vi "Render.vi"(8 "error in":errorcluster, 10 "Renderer in":refnum<class "Renderer.lvclass">, 11 "Dqmh Module":refnum<class "Dqmh Module.lvclass">) -> (0 "error out":errorcluster, 3 "Sections out":refnum<class "Section.lvclass">[](array[class]))   [LabVIEW 2021, in "TAF Proj Document Type.lvlib" / "Dqmh Module.lvclass"]
uses:
  <vilib>/Wovalab/AntiDoc/Document Type/Add-ons/LabVIEW TAF Project/Dqmh Module/Dqmh Module.lvclass
  C:/Program Files (x86)/National Instruments/LabVIEW 2021/vi.lib/Wovalab/AntiDoc/Bloc/Bloc.lvclass
  C:/Program Files (x86)/National Instruments/LabVIEW 2021/vi.lib/Wovalab/AntiDoc/Document Type/Add-ons/LabVIEW TAF Project/Lib/Lib.lvclass
  <vilib>/Wovalab/AntiDoc/Renderer/Renderer.lvclass
  <vilib>/Wovalab/AsciiDoc for LabVIEW/Section/Section.lvclass
  <vilib>/Wovalab/AsciiDoc for LabVIEW/Diagram/Type--enum.ctl
  <vilib>/Wovalab/AntiDoc/Document Type/Add-ons/LabVIEW TAF Project/Dqmh Module/Event Callers--cluster.ctl
  <vilib>/Wovalab/AsciiDoc for LabVIEW/Admonition/Types--enum.ctl
  <vilib>/Wovalab/AsciiDoc for LabVIEW/Table/Column Attributes--cluster.ctl
  <vilib>/Wovalab/AsciiDoc for LabVIEW/Table/Horizontal Alignment--enum.ctl
  <vilib>/Wovalab/AsciiDoc for LabVIEW/Table/Vertical Alignment--enum.ctl
  <vilib>/Wovalab/AsciiDoc for LabVIEW/Table/Style--enum.ctl
  <vilib>/Wovalab/AntiDoc/Bloc/Bloc.lvclass/Bloc.ctl
  <vilib>/Wovalab/AntiDoc/Document Type/Add-ons/LabVIEW TAF Project/Dqmh Module/Dqmh Module.lvclass/Dqmh Module.ctl
  <vilib>/Wovalab/AntiDoc/Document Type/Add-ons/LabVIEW TAF Project/Lib/Lib.lvclass/Lib.ctl
  <vilib>/Wovalab/AntiDoc/Renderer/Renderer.lvclass/Renderer.ctl
  <vilib>/Wovalab/AsciiDoc for LabVIEW/Table/Table.lvclass/Table.ctl
  <vilib>/Wovalab/AntiDoc/Renderer/Read Image Folder Path.vi
  <vilib>/Wovalab/AntiDoc/Bloc/Read Name.vi
  <vilib>/Wovalab/AntiDoc/Document Type/Add-ons/LabVIEW TAF Project/Dqmh Module/Read Dqmh Module Type.vi
  <vilib>/Wovalab/AntiDoc/Document Type/Add-ons/LabVIEW TAF Project/Lib/Read Description.vi
  <vilib>/Wovalab/AntiDoc/Document Type/Add-ons/LabVIEW TAF Project/Dqmh Module/Read Start Module Callers.vi
  <vilib>/Wovalab/AntiDoc/Document Type/Add-ons/LabVIEW TAF Project/Dqmh Module/Read Stop Module Callers.vi
  <vilib>/Wovalab/AntiDoc/Document Type/Add-ons/LabVIEW TAF Project/Dqmh Module/Read Request Link.vi
  <vilib>/Wovalab/AntiDoc/Document Type/Add-ons/LabVIEW TAF Project/Dqmh Module/Read Request With Reply Links.vi
  <vilib>/Wovalab/AntiDoc/Document Type/Add-ons/LabVIEW TAF Project/Dqmh Module/Read Broadcast Link.vi
  <vilib>/Wovalab/AntiDoc/Document Type/Add-ons/LabVIEW TAF Project/Dqmh Module/Read Registred Broadcast.vi
  <vilib>/Wovalab/AntiDoc/Document Type/Add-ons/LabVIEW TAF Project/Dqmh Module/Read Used Requests.vi
  <vilib>/Wovalab/AntiDoc/Document Type/Add-ons/LabVIEW TAF Project/Dqmh Module/Read Used Requests With Reply.vi
  <vilib>/Wovalab/AntiDoc/Document Type/Add-ons/LabVIEW TAF Project/Dqmh Module/Read Custom Errors.vi
  <vilib>/Wovalab/AntiDoc/Document Type/Add-ons/LabVIEW TAF Project/Lib/Read Vis.vi
  <vilib>/Wovalab/AntiDoc/Document Type/Add-ons/LabVIEW TAF Project/Dqmh Module/Read List Default Event.vi
  <vilib>/Wovalab/AsciiDoc for LabVIEW/Paragraph/Paragraph.lvclass
  C:/Program Files (x86)/National Instruments/LabVIEW 2021/vi.lib/Wovalab/AsciiDoc for LabVIEW/Adoc-Bloc/Bloc.lvclass
  <vilib>/Wovalab/AsciiDoc for LabVIEW/Admonition/Admonition.lvclass
  <vilib>/Wovalab/AsciiDoc for LabVIEW/Table/Table.lvclass
  <vilib>/Wovalab/AsciiDoc for LabVIEW/Diagram/Diagram.lvclass
  <vilib>/Wovalab/AsciiDoc for LabVIEW/Sub Section/Sub Section.lvclass
  C:/Program Files (x86)/National Instruments/LabVIEW 2021/vi.lib/Wovalab/AsciiDoc for LabVIEW/Section/Section.lvclass
  <vilib>/Wovalab/AsciiDoc for LabVIEW/Section/Add Bloc (array).vi
  <vilib>/Wovalab/AsciiDoc for LabVIEW/Sub Section/Create Sub Section (array).vi
  <vilib>/Wovalab/AntiDoc/Document Type/Add-ons/LabVIEW TAF Project/Vi/Vi.lvclass
  <vilib>/Wovalab/AntiDoc/Utilities/Utilities.lvlib
  C:/Program Files (x86)/National Instruments/LabVIEW 2021/vi.lib/Wovalab/AsciiDoc for LabVIEW/Paragraph/Paragraph.lvclass
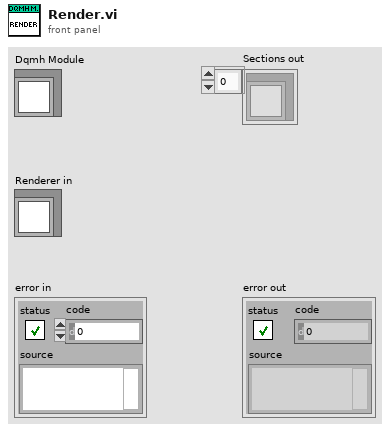
[diagram p1: front panel]
types:
  T1 = typedef "Wovalab_lib_AsciiDoctor.lvlib/Table.lvclass/Column Attributes--cluster.ctl" = cluster{"Width":u16, "Horizontal Alignment":T2, "Vertical Alignment":T3, "Style":T4}
  T2 = typedef "Wovalab_lib_AsciiDoctor.lvlib/Table.lvclass/Horizontal Alignment--enum.ctl" = enum16{"Left", "Center", "Right"}
  T3 = typedef "Wovalab_lib_AsciiDoctor.lvlib/Table.lvclass/Vertical Alignment--enum.ctl" = enum16{"Top", "Middle", "Bottom"}
  T4 = typedef "Wovalab_lib_AsciiDoctor.lvlib/Table.lvclass/Style--enum.ctl" = enum16{"None", "AsciiDoc", "Emphasis", "Header", "Literal", "Monospaced", "Strong", "Verse"}
  T5 = typedef "Wovalab_lib_AsciiDoctor.lvlib/Admonition.lvclass/Types--enum.ctl" = enum16{"Note", "Tip", "Important", "Warning", "Caution"}
  T6 = typedef "Wovalab_lib_AsciiDoctor.lvlib/Diagram.lvclass/Type--enum.ctl" = enum16{"a2s", "actdiag", "blockdiag", "ditaa", "erd", "graphviz", "meme", "mermaid", "msc", "nwdiag", "packetdiag", "plantuml", "rackdiag", "seqdiag", "shaape", "svgbob", "syntrax", "umlet", "vega", "vegalite", "wavedrom"}
  T7 = typedef "TAF Proj Document Type.lvlib/Dqmh Module.lvclass/Event Callers--cluster.ctl" = cluster{"Event Name":string, "Caller Names":string[]}
  T8 = typedef "TAF Proj Document Type.lvlib/Project Parser.lvlib/Dqmh Module Type--enum.ctl" = enum16{"Singleton", "Cloneable"}
  T9 = typedef "TAF Proj Document Type.lvlib/Dqmh Module.lvclass/Module Broadcast Registred--cluster.ctl" = cluster{"Module Name":string, "Registred Broadcasts":string[]}
  T10 = typedef "TAF Proj Document Type.lvlib/Dqmh Module.lvclass/Requests Used By Module--cluster.ctl" = cluster{"Module Name":string, "Request Names":string[]}
  T11 = typedef "AntiDoc.lvlib/Bloc.lvclass/Raw Custom Error Info--cluster.ctl" = cluster{"Code":i32, "Name":string, "Description":string, "Owned by":string}
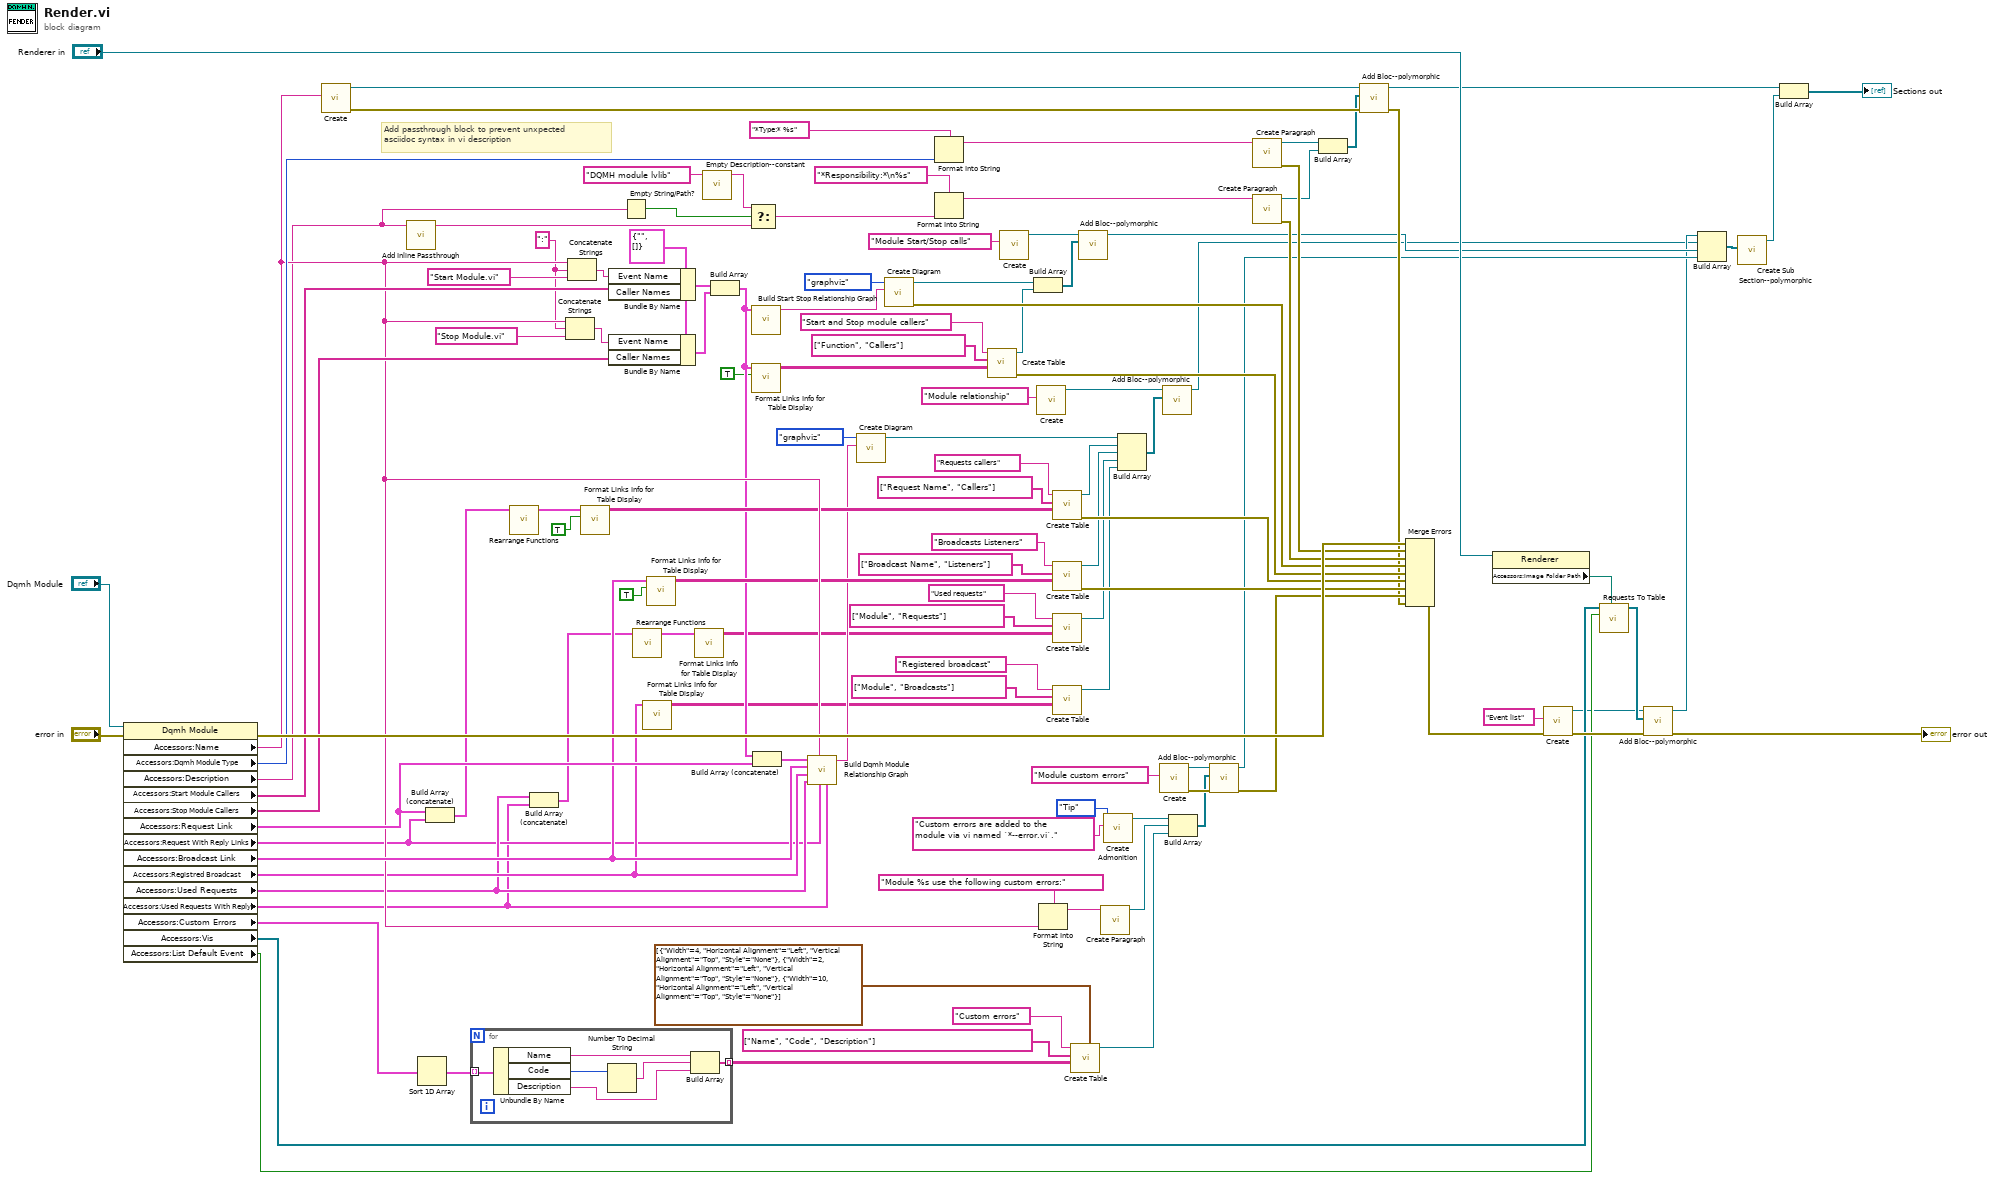
[diagram p0: block diagram]
diagram:
  w61 = T7 {"Event Name"="", "Caller Names"=[]} ("Request Callers")
  w69 = ":" ("string")
  # "Add passthrough block to prevent unxpected asciidoc syntax in vi description"
  n1 = property class="Dqmh Module"(reference="Dqmh Module", error in="error in") -> (error out=w119:errorcluster, "Accessors:Name"=w98:string, "Accessors:Dqmh Module Type"=w104:T8, "Accessors:Description"=w9:string, "Accessors:Start Module Callers"=w101:string[], "Accessors:Stop Module Callers"=w100:string[], "Accessors:Request Link"=w103:T7[], "Accessors:Request With Reply Links"=w91:T7[], "Accessors:Broadcast Link"=w102:T7[], "Accessors:Registred Broadcast"=w96:T9[], "Accessors:Used Requests"=w95:T10[], "Accessors:Used Requests With Reply"=w90:T10[], "Accessors:Custom Errors"=w94:T11[], "Accessors:Vis"=w93:refnum<class "Vi.lvclass">[], "Accessors:List Default Event"=w92:bool)  [unwired: 1 out]
  n2 = call <vilib>:"Create.vi"("Title"=w98) -> ("error out"=w118:errorcluster, "Section out"=w99:refnum<class "Section.lvclass">)  [unwired: 9 in]
  n3 = call <vilib>:"Add Inline Passthrough.vi"("String in"=w9) -> ("String out"=w8:string)  [unwired: 10 in]
  n4 = Sort 1D Array(array=w94) -> (sorted array=w22:T11[])
  n5 = Build Array (concatenate)(w103, w91) -> (w18:T7[])
  n6 = for {
    tunnel: w22 -> [w126] mode=indexing
    tunnel: [w122] -> w26 mode=indexing
    n7 = Unbundle By Name(w126) -> ("Name"=w125:string, "Code"=w121:i32, "Description"=w123:string)
    n8 = Number To Decimal String(number=w121) -> (decimal integer string=w124:string)  [unwired: 1 in]
    n9 = Build Array(w125, w124, w123) -> (w122:string[])
  }
  n10 = call <vilib>:"Rearrange Functions.vi"("Functions in"=w18) -> ("Functions in"=w17:T10[])  [unwired: 10 in]
  n11 = Build Array (concatenate)(w95, w90) -> (w20:T10[])
  n12 = Concatenate Strings(w98, w69, "Stop Module.vi" ("String")) -> (w67:string)
  n13 = Concatenate Strings(w98, w69, "Start Module.vi" ("String")) -> (w71:string)
  n14 = call <vilib>:"Format Links Info for Table Display.vi"("Remove module Name From First Column (F)"=TRUE ("Remove module Name From First Column"), "Links Info"=w17) -> ("Table Content"=w76:string[][])  [unwired: 9 in]
  n15 = Bundle By Name(cluster=w61, "Event Name"=w71, "Caller Names"=w101) -> (w66:T7)
  n16 = Bundle By Name(cluster=w61, "Event Name"=w67, "Caller Names"=w100) -> (w65:T7)
  n17 = Empty String/Path?(string/path=w9) -> (empty?=w85:bool)
  n18 = call <vilib>:"Rearrange Functions.vi"("Functions in"=w20) -> ("Functions in"=w19:T10[])  [unwired: 10 in]
  n19 = call <vilib>:"Format Links Info for Table Display.vi"("Links Info"=w96) -> ("Table Content"=w44:string[][])  [unwired: 10 in]
  n20 = call <vilib>:"Format Links Info for Table Display.vi"("Remove module Name From First Column (F)"=TRUE ("Remove module Name From First Column"), "Links Info"=w102) -> ("Table Content"=w75:string[][])  [unwired: 9 in]
  n21 = call <vilib>:"Format Links Info for Table Display.vi"("Links Info"=w19) -> ("Table Content"=w40:string[][])  [unwired: 10 in]
  n22 = call <vilib>:"Empty Description--constant.vi"("Description Source"="DQMH module lvlib") -> ("Empty Description"=w6:string)  [unwired: 10 in]
  n23 = Build Array(w66, w65) -> (w62:T7[])
  n24 = Select(t=w6, s=w85, f=w8) -> (s? t:f=w38:string)
  n25 = call <vilib>:"Build Start Stop Relationship Graph.vi"("Links Info"=w62) -> ("Graph"=w63:string)  [unwired: 10 in]
  n26 = call <vilib>:"Format Links Info for Table Display.vi"("Remove module Name From First Column (F)"=TRUE ("Remove module Name From First Column"), "Links Info"=w62) -> ("Table Content"=w72:string[][])  [unwired: 9 in]
  n27 = Build Array (concatenate)(w62, w103) -> (w60:T7[])
  n28 = call <vilib>:"Build Dqmh Module Relationship Graph.vi"("Used Requests With Reply"=w90, "Request With Reply Links Info"=w91, "Module Name"=w98, "Used Requests"=w95, "Registred Broadcast"=w96, "Broadcas Links Info"=w102, "Request Links Info"=w60) -> ("Graph"=w58:string)  [unwired: 4 in]
  n29 = call <vilib>:"Create Diagram.vi"("Diagram Source Code"=w58, "Diagram Type"=Type--enum."graphviz") -> ("Diagram out"=w50:refnum<class "Diagram.lvclass">)  [unwired: 8 in, 1 out]
  n30 = call <vilib>:"Create Diagram.vi"("Diagram Source Code"=w63, "Diagram Type"=Type--enum."graphviz") -> ("error out"=w111:errorcluster, "Diagram out"=w55:refnum<class "Diagram.lvclass">)  [unwired: 8 in]
  n31 = Format Into String(format string="*Responsibility:*\n%s", w38) -> (resulting string=w37:string)  [unwired: 2 in, 1 out]
  n32 = Format Into String(format string="*Type:* %s", w104) -> (resulting string=w80:string)  [unwired: 2 in, 1 out]
  n33 = call <vilib>:"Create Table.vi"("Content"=w72, "Header"=string[] ["Function", "Callers"], "Title"="Start and Stop module callers") -> ("error out"=w110:errorcluster, "Table out"=w54:refnum<class "Table.lvclass">)  [unwired: 7 in]
  n34 = call <vilib>:"Create.vi"("Title"="Module Start/Stop calls") -> ("Section out"=w56:refnum<class "Section.lvclass">)  [unwired: 9 in, 1 out]
  n35 = Build Array(w55, w54) -> (w53:refnum<class "Bloc.lvclass">[])
  n36 = call <vilib>:"Create.vi"("Title"="Module relationship") -> ("Section out"=w52:refnum<class "Section.lvclass">)  [unwired: 9 in, 1 out]
  n37 = Format Into String(format string="Module %s use the following custom errors:" ("Content"), w98) -> (resulting string=w27:string)  [unwired: 2 in, 1 out]
  n38 = call <vilib>:"Create Table.vi"("Content"=w76, "Header"=string[] ["Request Name", "Callers"], "Title"="Requests callers") -> ("error out"=w113:errorcluster, "Table out"=w49:refnum<class "Table.lvclass">)  [unwired: 7 in]
  n39 = call <vilib>:"Create Table.vi"("Content"=w75, "Header"=string[] ["Broadcast Name", "Listeners"], "Title"="Broadcasts Listeners") -> ("error out"=w112:errorcluster, "Table out"=w48:refnum<class "Table.lvclass">)  [unwired: 7 in]
  n40 = call <vilib>:"Create Table.vi"("Content"=w40, "Header"=string[] ["Module", "Requests"], "Title"="Used requests") -> ("Table out"=w39:refnum<class "Table.lvclass">)  [unwired: 7 in, 1 out]
  n41 = call <vilib>:"Create Table.vi"("Content"=w44, "Header"=string[] ["Module", "Broadcasts"], "Title"="Registered broadcast") -> ("Table out"=w43:refnum<class "Table.lvclass">)  [unwired: 7 in, 1 out]
  n42 = call <vilib>:"Create Table.vi"("Column Attributes"=T1[] [{"Width"=4, "Horizontal Alignment"=enum."Left", "Vertical Alignment"=enum."Top", "Style"=enum."None"}, {"Width"=2, "Horizontal Alignment"=enum."Left", "Vertical Alignment"=enum."Top", "Style"=enum."None"}, {"Width"=10, "Horizontal Alignment"=enum."Left", "Vertical Alignment"=enum."Top", "Style"=enum."None"}], "Content"=w26, "Header"=string[] ["Name", "Code", "Description"], "Title"="Custom errors") -> ("Table out"=w31:refnum<class "Table.lvclass">)  [unwired: 6 in, 1 out]
  n43 = call-poly <vilib>:"Add Bloc--polymorphic.vi"("Bloc"=w53, "Section in"=w56) -> ("Section out"=w5:refnum<class "Section.lvclass">)  [unwired: 8 in, 1 out]
  n44 = call <vilib>:"Create Paragraph.vi"("Content"=w27) -> ("Paragraph out"=w29:refnum<class "Paragraph.lvclass">)  [unwired: 9 in, 1 out]
  n45 = call <vilib>:"Create Admonition.vi"("Content"="Custom errors are added to the module via vi named `*--error.vi`.", "Types"=Types--enum."Tip") -> ("Admonition out"=w23:refnum<class "Admonition.lvclass">)  [unwired: 8 in, 1 out]
  n46 = Build Array(w50, w49, w48, w39, w43) -> (w47:refnum<class "Bloc.lvclass">[])
  n47 = call <vilib>:"Create.vi"("Title"="Module custom errors") -> ("error out"=w109:errorcluster, "Section out"=w34:refnum<class "Section.lvclass">)  [unwired: 9 in]
  n48 = call-poly <vilib>:"Add Bloc--polymorphic.vi"("Bloc"=w47, "Section in"=w52) -> ("Section out"=w2:refnum<class "Section.lvclass">)  [unwired: 8 in, 1 out]
  n49 = Build Array(w23, w29, w31) -> (w30:refnum<class "Bloc.lvclass">[])
  n50 = call-poly <vilib>:"Add Bloc--polymorphic.vi"("error in"=w109, "Bloc"=w30, "Section in"=w34) -> ("error out"=w108:errorcluster, "Section out"=w4:refnum<class "Section.lvclass">)  [unwired: 7 in]
  n51 = call <vilib>:"Create Paragraph.vi"("Content"=w80) -> ("error out"=w115:errorcluster, "Paragraph out"=w81:refnum<class "Paragraph.lvclass">)  [unwired: 9 in]
  n52 = call <vilib>:"Create Paragraph.vi"("Content"=w37) -> ("error out"=w114:errorcluster, "Paragraph out"=w86:refnum<class "Paragraph.lvclass">)  [unwired: 9 in]
  n53 = Build Array(w81, w86) -> (w84:refnum<class "Paragraph.lvclass">[])
  n54 = call-poly <vilib>:"Add Bloc--polymorphic.vi"("error in"=w118, "Bloc"=w84, "Section in"=w99) -> ("error out"=w107:errorcluster, "Section out"=w88:refnum<class "Section.lvclass">)  [unwired: 7 in]
  n55 = Merge Errors(w119, w115, w114, w111, w110, w113, w112, w108, w107) -> (w116:errorcluster)
  n56 = property class="Renderer"(reference="Renderer in") -> ("Accessors:Image Folder Path"=w12:path)  [unwired: 1 in, 2 out]
  n57 = call <vilib>:"Create.vi"("error in (no error)"=w116, "Title"="Event list") -> ("error out"=w106:errorcluster, "Section out"=w10:refnum<class "Section.lvclass">)  [unwired: 8 in]
  n58 = call <vilib>:"Requests To Table.vi"("Image Folder Path"=w12, "List Default Event"=w92, "Dqmh Events"=w93) -> ("Table"=w13:refnum<class "Bloc.lvclass">[])  [unwired: 8 in]
  n59 = call-poly <vilib>:"Add Bloc--polymorphic.vi"("error in"=w106, "Bloc"=w13, "Section in"=w10) -> ("error out"=→"error out":errorcluster, "Section out"=w3:refnum<class "Section.lvclass">)  [unwired: 7 in]
  n60 = Build Array(w3, w2, w5, w4) -> (w1:refnum<class "Section.lvclass">[])
  n61 = call-poly <vilib>:"Create Sub Section--polymorphic.vi"("Section"=w1) -> ("Sub Section out"=w87:refnum<class "Sub Section.lvclass">)  [unwired: 9 in, 1 out]
  n62 = Build Array(w88, w87) -> (→"Sections out":refnum<class "Section.lvclass">[])
